vi "Set Controls Disable (all).vi"(8 "error in (no error)":errorcluster, 10 "disable state":T2(ring), 11 "control references":T1) -> (0 "error out":errorcluster)   [LabVIEW 2017]
uses:
  Controls/Error Codes List Window References.ctl
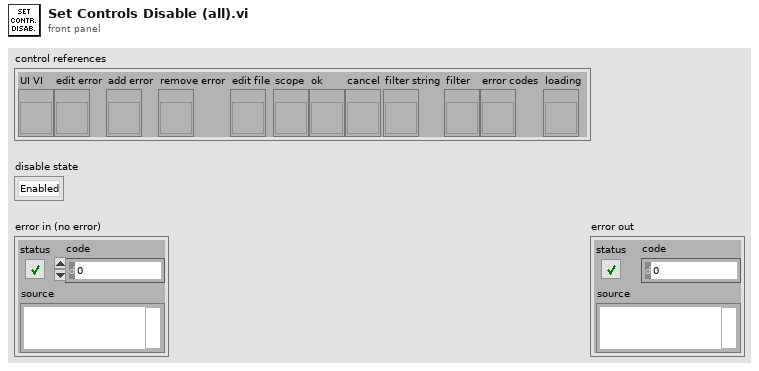
[diagram p1: front panel]
types:
  T1 = typedef "Error Codes List Window References.ctl" = cluster{"UI VI":refnum<vi>, "edit error":refnum<vi>, "add error":refnum<vi>, "remove error":refnum<vi>, "edit file":refnum<vi>, "scope":refnum<vi>, "ok":refnum<vi>, "cancel":refnum<vi>, "filter string":refnum<vi>, "filter":refnum<vi>, "error codes":refnum<vi>, "loading":refnum<vi>}
  T2 = enum8{"Enabled", "Disabled", "Disabled and Grayed Out"}
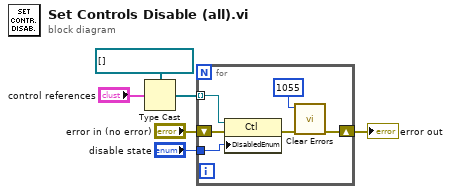
[diagram p0: block diagram]
diagram:
  n1 = Type Cast(type=refnum<vi>[] [] ("edit error"), x="control references") -> (*(type *) &x=w3:refnum<vi>[])
  n2 = for {
    tunnel: w3 -> [w9] mode=indexing
    tunnel: "disable state" -> [w12]
    shift-right: [w8] -> w6
    shift-left: "error in (no error)" -> [w11]
    n3 = property on="Property Node" class="Ctl"(reference=w9, error in=w11, "DisabledEnum"=w12) -> (error out=w10:errorcluster)  [unwired: 1 out]
    n4 = call <vilib>:"Clear Errors.vi"("error in (no error)"=w10, "specific error code to clear (0: all)"=1055) -> ("error out"=w8:errorcluster)  [unwired: 4 in, 1 out]
  }
  "error out" <- w6
